vi "snr_all_in_one.vi"(8 "error in (no error)":errorcluster, 10 "controls":T2={"snr window width [Hz]"=20.0, "harmonic N"=0, "start time"=0.0, "Sec"=0.0, "resolution windows duration"=20.0}, 11 "waveform":waveform(dbl)) -> (0 "error out":errorcluster, 3 "output cluster":T1)   [LabVIEW 2019]
uses:
  <vilib>/Analysis/1siggen.llb/Ramp Pattern by Delta.vi
  <vilib>/Analysis/NI_AALBase.lvlib
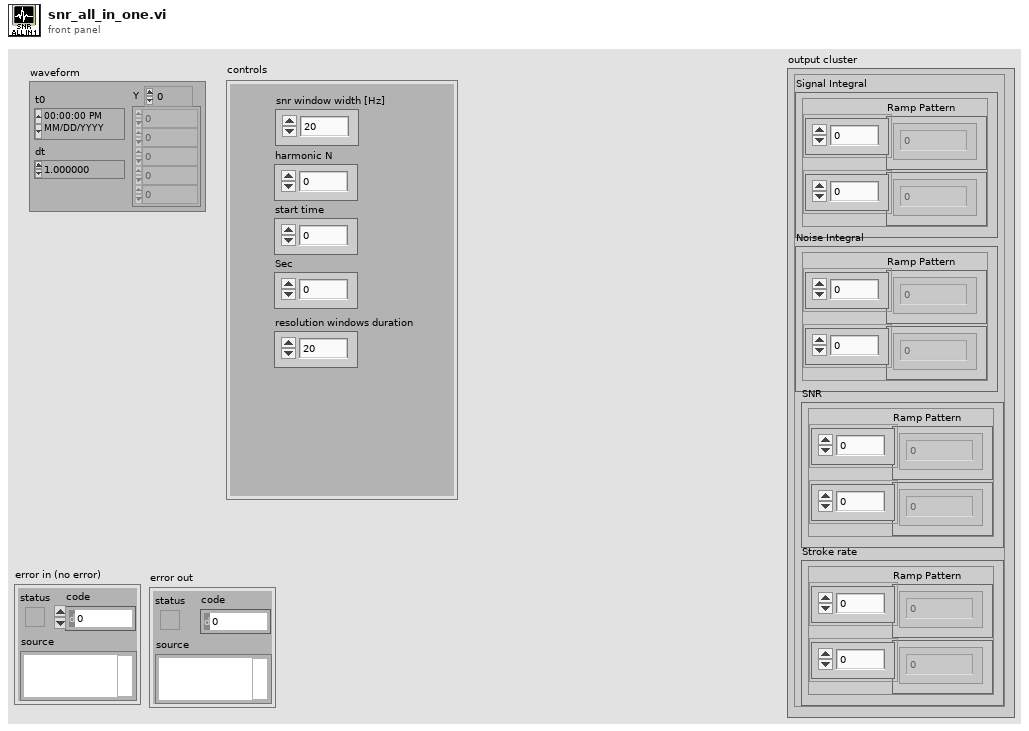
[diagram p1: front panel]
types:
  T1 = cluster{"Signal Integral":cluster{"Ramp Pattern":dbl[], "Array":dbl[]}, "Noise Integral":cluster{"Ramp Pattern":dbl[], "Array":dbl[]}, "SNR":cluster{"Ramp Pattern":dbl[], "Array":dbl[]}, "Stroke rate":cluster{"Ramp Pattern":dbl[], "Array":dbl[]}}
  T2 = cluster{"snr window width [Hz]":dbl, "harmonic N":i32, "start time":dbl, "Sec":dbl, "resolution windows duration":dbl}
  T3 = cluster{"start samples/time":dbl, "duration":dbl, "snr window width [Hz]":dbl, "harmonic N":i32}
  T4 = cluster{"Signal Integral":dbl, "Noise Integral":dbl, "SNR":dbl, "PSD":cluster{"f0":dbl, "df":dbl, "magnitude":dbl[]}[], "Amplitude":dbl, "Frequency":dbl, "Stroke rate [stroke/min]":dbl}
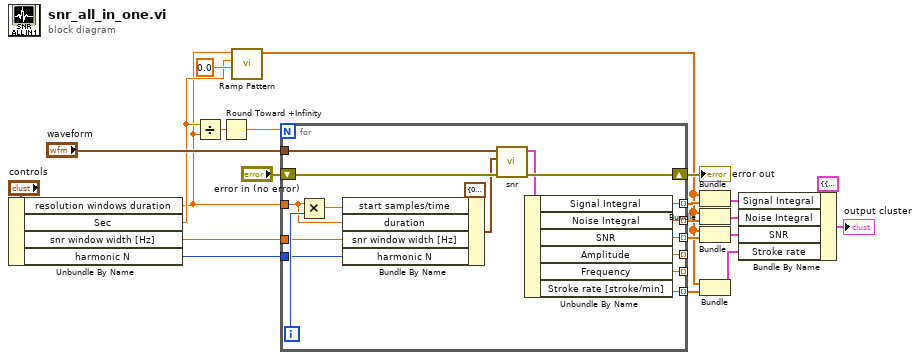
[diagram p0: block diagram]
diagram:
  n1 = Unbundle By Name("controls") -> ("resolution windows duration"=w13:dbl, "Sec"=w14:dbl, "snr window width [Hz]"=w17:dbl, "harmonic N"=w16:i32)
  n2 = Divide(x=w14, y=w13) -> (x/y=w19:dbl)
  n3 = Round Toward +Infinity(x=w19) -> (ceil(x): smallest int >= x=w1:dbl)
  n4 = call-poly <vilib>:"Ramp Pattern.vi"("start"=0.0, "end"=w14, "delta"=w13) -> ("Ramp Pattern"=w8:dbl[])  [unwired: 6 in, 2 out]
  n5 = for {
    N: w1 -> [_]
    tunnel: "waveform" -> [w39]
    shift-right: [w37] -> w20
    shift-left: "error in (no error)" -> [w38]
    tunnel: w13 -> [w32]
    tunnel: w17 -> [w31]
    tunnel: w16 -> [w30]
    tunnel: [w28] -> w11 mode=indexing
    tunnel: [w27] -> w12 mode=indexing
    tunnel: [w26] -> w10 mode=indexing
    tunnel: [w25] -> _ mode=indexing
    tunnel: [w24] -> _ mode=indexing
    tunnel: [w23] -> w9 mode=indexing
    i -> [w34]
    n6 = Multiply(x=w32, y=w34) -> (x*y=w33:dbl)
    n7 = Bundle By Name(cluster=T3 {"start samples/time"=0.0, "duration"=0.0, "snr window width [Hz]"=0.0, "harmonic N"=0} ("snr config"), "start samples/time"=w33, "duration"=w32, "snr window width [Hz]"=w31, "harmonic N"=w30) -> (w35:T3)
    n8 = call "snr.vi"("error in (no error)"=w38, "snr config"=w35, "waveform"=w39) -> ("error out"=w37:errorcluster, "SNR data"=w29:T4)  [unwired: 7 in]
    n9 = Unbundle By Name(w29) -> ("Signal Integral"=w27:dbl, "Noise Integral"=w28:dbl, "SNR"=w26:dbl, "Amplitude"=w25:dbl, "Frequency"=w24:dbl, "Stroke rate [stroke/min]"=w23:dbl)
  }
  "error out" <- w20
  n10 = Bundle("Ramp Pattern"=w8, w12) -> (w7:cluster{"Ramp Pattern":dbl[], dbl[]})  [unwired: 1 in]
  n11 = Bundle("Ramp Pattern"=w8, w11) -> (w6:cluster{"Ramp Pattern":dbl[], dbl[]})  [unwired: 1 in]
  n12 = Bundle("Ramp Pattern"=w8, w10) -> (w5:cluster{"Ramp Pattern":dbl[], dbl[]})  [unwired: 1 in]
  n13 = Bundle("Ramp Pattern"=w8, w9) -> (w4:cluster{"Ramp Pattern":dbl[], dbl[]})  [unwired: 1 in]
  n14 = Bundle By Name(cluster=T1 {"Signal Integral"={"Ramp Pattern"=[], "Array"=[]}, "Noise Integral"={"Ramp Pattern"=[], "Array"=[]}, "SNR"={"Ramp Pattern"=[], "Array"=[]}, "Stroke rate"={"Ramp Pattern"=[], "Array"=[]}} ("output cluster"), "Signal Integral"=w7, "Noise Integral"=w6, "SNR"=w5, "Stroke rate"=w4) -> (→"output cluster":T1)
